vi "Waveforms.Close.vi"(8 "error in (no error)":errorcluster, 11 "Waveforms":T5) -> (0 "error out":errorcluster)   [LabVIEW 2019]
uses:
  <vilib>/NI VeriStand/Execution/WaveformStreaming/WaveformStreamSpecification.ctl
  NationalInstruments.VeriStand.ClientAPI
  <vilib>/NI VeriStand/Execution/WaveformStreaming/Registered Waveform Streams Data Event Refnum (DBL).ctl
  <vilib>/NI VeriStand/Execution/WaveformStreaming/Waveform Data Watcher Event Data (DBL).ctl
  <vilib>/NI VeriStand/Execution/WaveformStreaming/WaveformDataWatcherDBL.ctl
  <vilib>/NI VeriStand/Execution/WaveformStreaming/WaveformStreamingAPI.ctl
  <vilib>/NI VeriStand/Execution/WaveformStreaming/Unregister for Waveform Data Events (DBL).vi
  <vilib>/NI VeriStand/Execution/WaveformStreaming/NI_VS Waveform Streaming Interface.lvlib
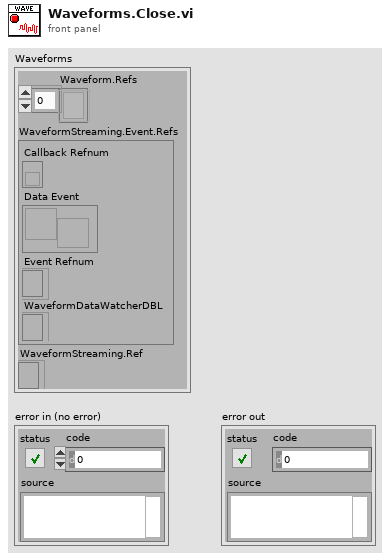
[diagram p1: front panel]
types:
  T1 = typedef "NI_VS Waveform Streaming Interface.lvlib/WaveformStreamSpecification.ctl" = refnum<k24>
  T2 = typedef "NI_VS Waveform Streaming Interface.lvlib/Registered Waveform Streams Data Event Refnum (DBL).ctl" = cluster{"Callback Refnum":refnum<k27>, "Data Event":refnum<user-event>, "Event Refnum":refnum<event-registration>, "WaveformDataWatcherDBL":T3}
  T3 = typedef "NI_VS Waveform Streaming Interface.lvlib/WaveformDataWatcherDBL.ctl" = refnum<k24>
  T4 = typedef "NI_VS Waveform Streaming Interface.lvlib/WaveformStreamingAPI.ctl" = refnum<k24>
  T5 = cluster{"Waveform.Refs":T1[], "WaveformStreaming.Event.Refs":T2, "WaveformStreaming.Ref":T4}
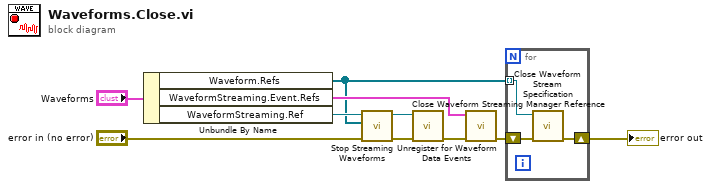
[diagram p0: block diagram]
diagram:
  n1 = Unbundle By Name("Waveforms") -> ("Waveform.Refs"=w8:T1[], "WaveformStreaming.Event.Refs"=w10:T2, "WaveformStreaming.Ref"=w9:T4)
  n2 = call <vilib>:"Stop Streaming Waveforms.vi"("error in (no error)"="error in (no error)", "WaveformStreamSpecifications"=w8, "WaveformStreaming in"=w9) -> ("error out"=w2:errorcluster, "WaveformStreaming out"=w3:T4)  [unwired: 7 in]
  n3 = call <vilib>:"Close Waveform Streaming Manager Reference.vi"("error in (no error)"=w2, "WaveformStreaming"=w3) -> ("error out"=w4:errorcluster)  [unwired: 9 in]
  n4 = call-poly <vilib>:"Unregister for Waveform Data Events.vi"("error in (no error)"=w4, "registered waveform data event (DBL)"=w10) -> ("error out"=w5:errorcluster)  [unwired: 9 in]
  n5 = for {
    shift-right: [w12] -> w6
    shift-left: w5 -> [w13]
    tunnel: w8 -> [w11] mode=indexing
    n6 = call <vilib>:"Close Waveform Stream Specification.vi"("error in (no error)"=w13, "WaveformStreamSpecification"=w11) -> ("error out"=w12:errorcluster)  [unwired: 9 in]
  }
  "error out" <- w6
